vi "Set Dev Rolloff.vi"(8 "error in (no error)":errorcluster, 9 "firmware revision":string(combo), 10 "dev rolloff (3000)":dbl=3000.0, 11 "VISA resource name":refnum<visa-resource-name>) -> (0 "error out":errorcluster, 2 "bridge error":T1, 3 "VISA resource name out":refnum<visa-resource-name>)   [LabVIEW 2020, in "Andeen-Hagerling 2700A.lvlib"]
doc: "Sets the 3 db down point of the analog output frequency roll\noff limit."
uses:
  Andeen-Hagerling 2700A.lvlib
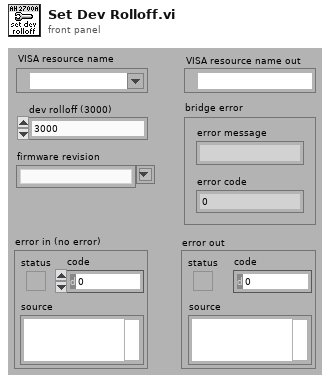
[diagram p1: front panel]
types:
  T1 = cluster{"error message":string, "error code":i32}
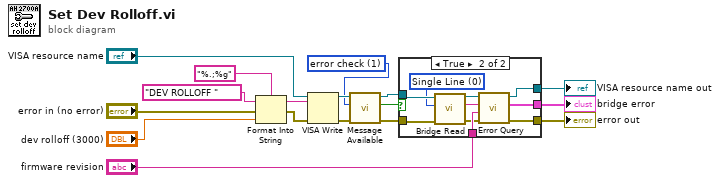
[diagram p0: block diagram]
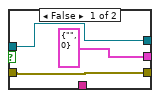
[diagram p2: hidden frame]
diagram:
  w1 = u16 1 items=["none", "error check", "multiline read", "infinite"] ("delay")
  n1 = Format Into String(format string="%.;%g", initial string="DEV ROLLOFF " ("command"), error in="error in (no error)", "dev rolloff (3000)") -> (resulting string=w13:string, error out=w14:errorcluster)
  n2 = VISA Write(VISA resource name="VISA resource name", write buffer=w13, error in (no error)=w14) -> (VISA resource name out=w6:refnum<visa-resource-name>, error out=w5:errorcluster)  [unwired: 1 out]
  n3 = call "Message Available.vi"("error in (no error)"=w5, "delay"=w1, "VISA resource name"=w6) -> ("error out"=w8:errorcluster, "message available"=w10:bool, "VISA resource name out"=w9:refnum<visa-resource-name>)  [unwired: 6 in]
  n4 = case shown="True" w10 {
    tunnel: w9 -> [w19 w23]
    tunnel: w8 -> [w20 w22]
    tunnel: "firmware revision" -> [_ w30]
    tunnel: [w20 w29] -> w4
    tunnel: [w19 w28] -> w3
    tunnel: [T1 {"error message"="", "error code"=0} ("bridge error") w27] -> w2
    frame False {
    }
    frame True {
      w21 = u16 0 items=["Single Line", "Multi-Line"] ("Multiline")
      n5 = call "Bridge Read.vi"("error in (no error)"=w22, "multiline"=w21, "VISA resource name"=w23) -> ("error out"=w24:errorcluster, "read buffer"=w25:string, "VISA resource name out"=w26:refnum<visa-resource-name>)  [unwired: 6 in]
      n6 = call "Error Query.vi"("error in (no error)"=w24, "firmware revision"=w30, "measurement line"=w25, "VISA resource name"=w26) -> ("error out"=w29:errorcluster, "bridge error"=w27:T1, "VISA resource name out"=w28:refnum<visa-resource-name>)  [unwired: 5 in]
    }
  }
  "VISA resource name out" <- w3
  "error out" <- w4
  "bridge error" <- w2
